vi "get_readiness.vi"(8 "error in (no error)":errorcluster, 11 "DAQ_DL090211Scaffold in":refnum<class "DAQ_DL090211Scaffold.lvclass">) -> (0 "error out":errorcluster, 2 "ready?":bool, 3 "DAQ_DL090211Scaffold out":refnum<class "DAQ_DL090211Scaffold.lvclass">)   [LabVIEW 2010, in "DAQ_DL090211Scaffold.lvclass"]
uses:
  DAQ_DL090211Scaffold.lvclass
  DAQ_DL090211Scaffold.lvclass/DAQ_DL090211Scaffold.ctl
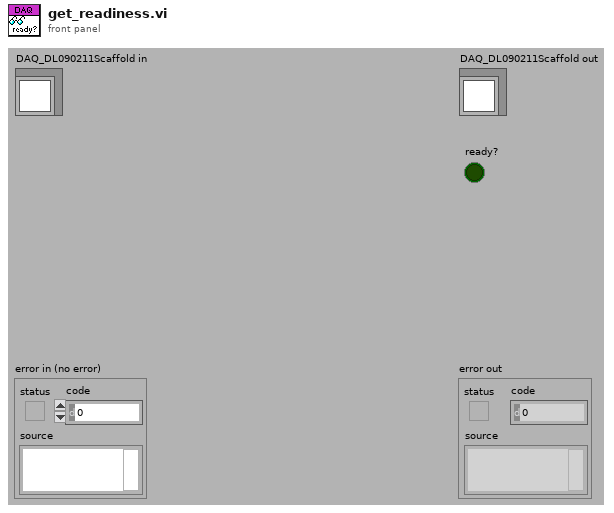
[diagram p1: front panel]
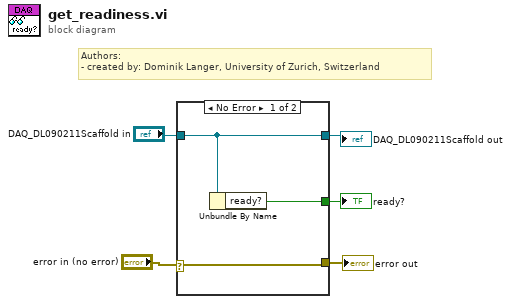
[diagram p0: block diagram]
diagram:
  # "Authors: \n- created by: Dominik Langer, University of Zurich, Switzerland"
  n1 = case shown="No Error" "error in (no error)" {
    selector: "error in (no error)" -> [w8 w10]
    tunnel: [w8 w10] -> w4
    tunnel: [w7 _] -> w3
    tunnel: [w6 w9] -> w1
    tunnel: "DAQ_DL090211Scaffold in" -> [w6 w9]
    frame No Error {
      n2 = Unbundle By Name(w6) -> ("ready?"=w7:bool)
    }
    frame Error {
    }
  }
  "error out" <- w4
  "DAQ_DL090211Scaffold out" <- w1
  "ready?" <- w3
